vi "oa_SCL Calc Inner Rect.vi"(1 "grid cosmetics":T2={"line color"=39168, "text color"=65280, "tick length"=3, "crossing axes"=FALSE, "visible grid?"=TRUE}, 2 "y text rect":T1, 3 "x text rect":T1, 4 "graph rect":T1) -> (0 "inner rect":T1)   [LabVIEW 2017]
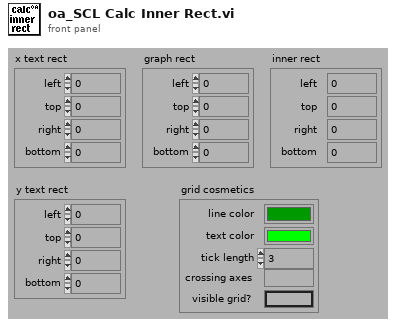
[diagram p1: front panel]
types:
  T1 = cluster{"left":i16, "top":i16, "right":i16, "bottom":i16}
  T2 = cluster{"line color":u32, "text color":u32, "tick length":i16, "crossing axes":bool, "visible grid?":bool}
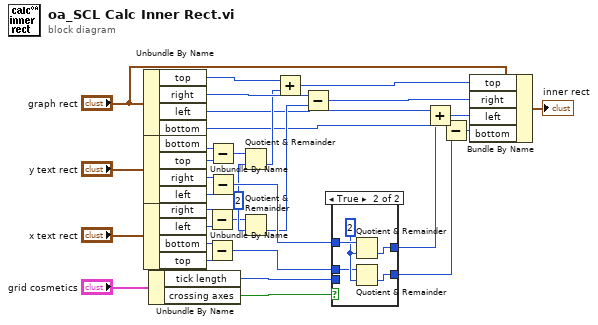
[diagram p0: block diagram]
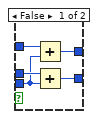
[diagram p2: hidden frame]
diagram:
  w12 = i16 2
  n1 = Unbundle By Name("graph rect") -> ("top"=w8:i16, "right"=w9:i16, "left"=w4:i16, "bottom"=w3:i16)
  n2 = Unbundle By Name("y text rect") -> ("bottom"=w31:i16, "top"=w30:i16, "right"=w29:i16, "left"=w28:i16)
  n3 = Unbundle By Name("x text rect") -> ("right"=w24:i16, "left"=w25:i16, "bottom"=w26:i16, "top"=w27:i16)
  n4 = Unbundle By Name("grid cosmetics") -> ("tick length"=w21:i16, "crossing axes"=w19:bool)
  n5 = Subtract(x=w24, y=w25) -> (x-y=w11:i16)
  n6 = Subtract(x=w26, y=w27) -> (x-y=w18:i16)
  n7 = Subtract(x=w31, y=w30) -> (x-y=w17:i16)
  n8 = Subtract(x=w29, y=w28) -> (x-y=w16:i16)
  n9 = Quotient & Remainder(x=w17, y=w12) -> (floor(x/y)=w7:i16)  [unwired: 1 out]
  n10 = Quotient & Remainder(x=w11, y=w12) -> (floor(x/y)=w10:i16)  [unwired: 1 out]
  n11 = Add(x=w8, y=w7) -> (x+y=w15:i16)
  n12 = Subtract(x=w9, y=w10) -> (x-y=w14:i16)
  n13 = case shown="True" w19 {
    tunnel: w16 -> [w34 w42]
    tunnel: w21 -> [w33 _]
    tunnel: w18 -> [w37 w40]
    tunnel: [w36 w39] -> w2
    tunnel: [w35 w38] -> w1
    frame False {
      n14 = Add(x=w34, y=w33) -> (x+y=w36:i16)
      n15 = Add(x=w37, y=w33) -> (x+y=w35:i16)
    }
    frame True {
      w41 = i16 2
      n16 = Quotient & Remainder(x=w42, y=w41) -> (floor(x/y)=w39:i16)  [unwired: 1 out]
      n17 = Quotient & Remainder(x=w40, y=w41) -> (floor(x/y)=w38:i16)  [unwired: 1 out]
    }
  }
  n18 = Add(x=w4, y=w2) -> (x+y=w6:i16)
  n19 = Subtract(x=w3, y=w1) -> (x-y=w5:i16)
  n20 = Bundle By Name(cluster="graph rect", "top"=w15, "right"=w14, "left"=w6, "bottom"=w5) -> (→"inner rect":T1)
